vi "EnvMillikCheckChannels.vi"(7 "channel array in":string[](array[string]), 8 "error in (no error)":errorcluster, 9 "sensor id array in":i32[](array[numeric]), 10 "db connection in":T1, 11 "VISA Refnum in":refnum<visa-resource-name>) -> (0 "error out":errorcluster, 1 "sensor id array out":i32[](array[numeric]), 2 "db connection out":T1, 3 "VISA Refnum out":refnum<visa-resource-name>, 5 "channel array out":string[](array[string]))   [LabVIEW 2016]
uses:
  <vilib>/addons/database/Connection.llb/Conn ObjectReference.ctl
  <vilib>/addons/database/NI_Database_API.lvlib
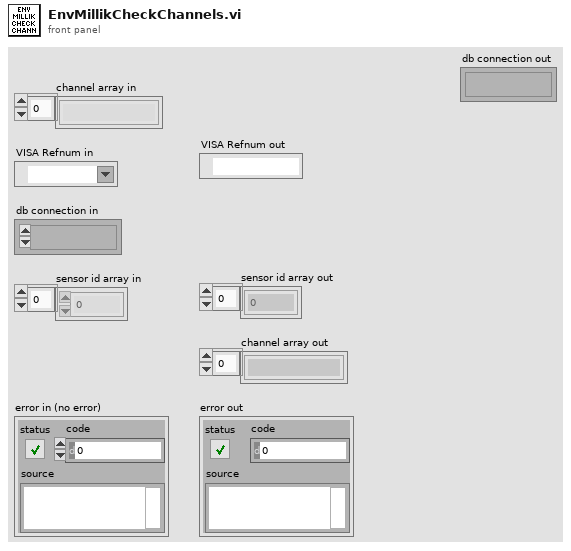
[diagram p1: front panel]
types:
  T1 = typedef "NI_Database_API.lvlib/Conn ObjectReference.ctl" = refnum<k1>
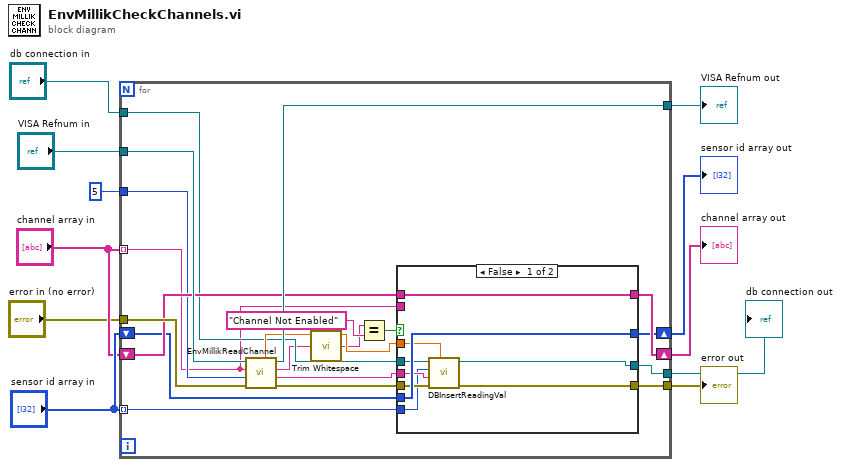
[diagram p0: block diagram]
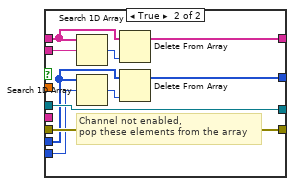
[diagram p2: hidden frame]
diagram:
  n1 = for {
    tunnel: "VISA Refnum in" -> [w29]
    tunnel: [w31] -> w5
    tunnel: "error in (no error)" -> [w30]
    tunnel: [w24] -> w3
    shift-right: [w23] -> w7
    shift-left: "channel array in" -> [w22]
    shift-right: [w20] -> w6
    shift-left: "sensor id array in" -> [w21]
    tunnel: "channel array in" -> [w12] mode=indexing
    tunnel: "sensor id array in" -> [w18] mode=indexing
    tunnel: "db connection in" -> [w17]
    tunnel: [w16] -> w1
    tunnel: 5 ("y") -> [w15]
    n2 = call "EnvMillikReadChannel.vi"("error in (no error)"=w30, "timeout"=w15, "channel"=w12, "VISA Refnum in"=w29) -> ("error out"=w25:errorcluster, "timestamp"=w19:string, "read buffer"=w14:string, "VISA Refnum out"=w31:refnum<visa-resource-name>, "value"=w26:dbl)  [unwired: 3 in]
    n3 = call <vilib>:"Trim Whitespace.vi"("string"=w14) -> ("trimmed string"=w13:string)  [unwired: 1 in]
    n4 = Equal?(x=w13, y="Channel Not Enabled") -> (x = y?=w27:bool)
    n5 = case shown="False" w27 {
      tunnel: w26 -> [w38 _]
      tunnel: w25 -> [w37 w47]
      tunnel: [w36 w47] -> w24
      tunnel: [w39 w50] -> w23
      tunnel: w22 -> [w39 w43]
      tunnel: w21 -> [w40 w46]
      tunnel: [w40 w49] -> w20
      tunnel: w19 -> [w35 _]
      tunnel: w18 -> [w34 w45]
      tunnel: w17 -> [w33 w48]
      tunnel: [w32 w48] -> w16
      tunnel: w12 -> [_ w42]
      frame False {
        n6 = call "DBInsertReadingVal.vi"("db connection in"=w33, "sensor id"=w34, "timestamp"=w35, "error in (no error)"=w37, "reading value"=w38) -> ("db connection out"=w32:T1, "error out"=w36:errorcluster)  [unwired: 4 in]
      }
      frame True {
        # "Channel not enabled, \npop these elements from the array"
        n7 = Search 1D Array(1D array=w43, element=w42) -> (index of element=w41:i32)  [unwired: 1 in]
        n8 = Search 1D Array(1D array=w46, element=w45) -> (index of element=w44:i32)  [unwired: 1 in]
        n9 = Delete From Array(array=w43, index=w41) -> (array with subset deleted=w50:string[])  [unwired: 1 in, 1 out]
        n10 = Delete From Array(array=w46, index=w44) -> (array with subset deleted=w49:i32[])  [unwired: 1 in, 1 out]
      }
    }
  }
  "channel array out" <- w7
  "sensor id array out" <- w6
  "VISA Refnum out" <- w5
  "error out" <- w3
  "db connection out" <- w1
